vi "Sets the ACW test frequency for MANU.vi"(5 "Enable to Query":bool, 7 "Enable to Setup":bool, 8 "error in":errorcluster, 10 "ACW Test Frequency(Hz)":u8(ring)=1 items=["50", "60"], 11 "VISA resource name":refnum<visa-resource-name>) -> (0 "error out":errorcluster, 2 "Return the ACW Test Frequency":string, 3 "VISA resource name out":refnum<visa-resource-name>)   [LabVIEW 2011, in "GPT-9000.lvlib"]
uses:
  <instrlib>/GPT-9000/GPT-9000.lvlib
panel:
  # "Hz"
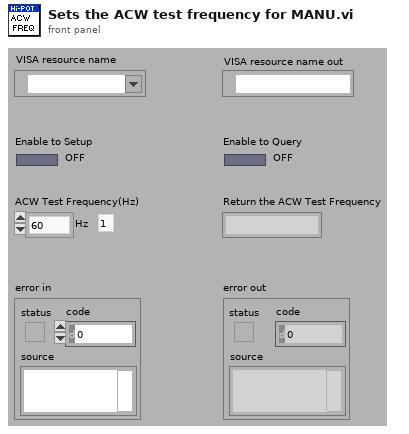
[diagram p1: front panel]
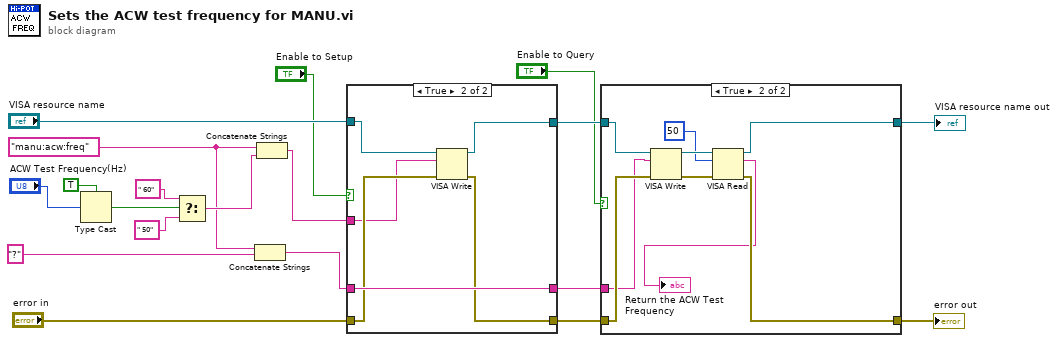
[diagram p0: block diagram]
diagram:
  w12 = "manu:acw:freq"
  n1 = Type Cast(type=TRUE, x="ACW Test Frequency(Hz)") -> (*(type *) &x=w15:bool)
  n2 = Select(t=" 60", s=w15, f=" 50") -> (s? t:f=w14:string)
  n3 = Concatenate Strings(w12, "?") -> (w10:string)
  n4 = Concatenate Strings(w12, w14) -> (w11:string)
  n5 = case shown="True" "Enable to Setup" {
    tunnel: w11 -> [_ w25]
    tunnel: w10 -> [w20 w28]
    tunnel: "VISA resource name" -> [w22 w27]
    tunnel: "error in" -> [w21 w26]
    tunnel: [w22 w24] -> w7
    tunnel: [w21 w23] -> w6
    tunnel: [w20 w28] -> w5
    frame False {
    }
    frame True {
      n6 = VISA Write(VISA resource name=w27, write buffer=w25, error in (no error)=w26) -> (VISA resource name out=w24:refnum<visa-resource-name>, error out=w23:errorcluster)  [unwired: 1 out]
    }
  }
  n7 = case shown="True" "Enable to Query" {
    tunnel: w7 -> [w30 w36]
    tunnel: w6 -> [w29 w35]
    tunnel: w5 -> [_ w34]
    tunnel: [w30 w33] -> w4
    tunnel: [w29 w32] -> w3
    frame False {
    }
    frame True {
      n8 = VISA Write(VISA resource name=w36, write buffer=w34, error in (no error)=w35) -> (VISA resource name out=w38:refnum<visa-resource-name>, error out=w39:errorcluster)  [unwired: 1 out]
      n9 = VISA Read(VISA resource name=w38, byte count=u32 50, error in (no error)=w39) -> (VISA resource name out=w33:refnum<visa-resource-name>, read buffer=→"Return the ACW Test Frequency":string, error out=w32:errorcluster)  [unwired: 1 out]
    }
  }
  "VISA resource name out" <- w4
  "error out" <- w3
